vi "__move_motor2.vi"(3 "Moving distance":dbl=-50.0, 5 "motor setup":T1={"Axis"=0, "ID"=0, "HIspeed"=100.0, "LOspeed"=100.0, "ACCEL(ms)"=100.0, "Sratio"=50.0, "free ride"=TRUE, "string"="DSB HOT/COLD"}) -> (0 "error out":errorcluster, 2 "counter":dbl)   [LabVIEW 2017]
panel:
  in  "Ball":bool
  in  "Mcsd":refnum<k7>(container)
  # "<= HOT = reset to 0 and reset"
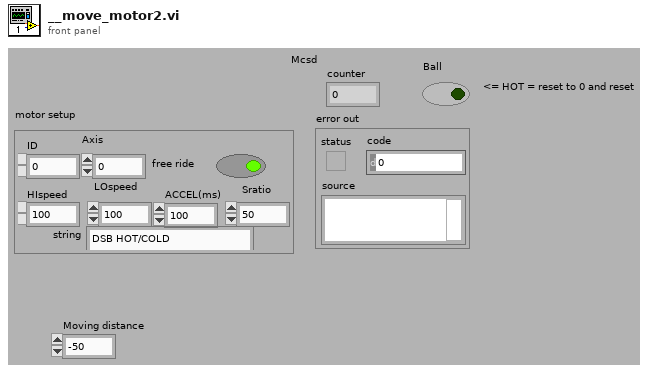
[diagram p1: front panel]
types:
  T1 = cluster{"Axis":i16, "ID":i16, "HIspeed":dbl, "LOspeed":dbl, "ACCEL(ms)":dbl, "Sratio":dbl, "free ride":bool, "string":string}
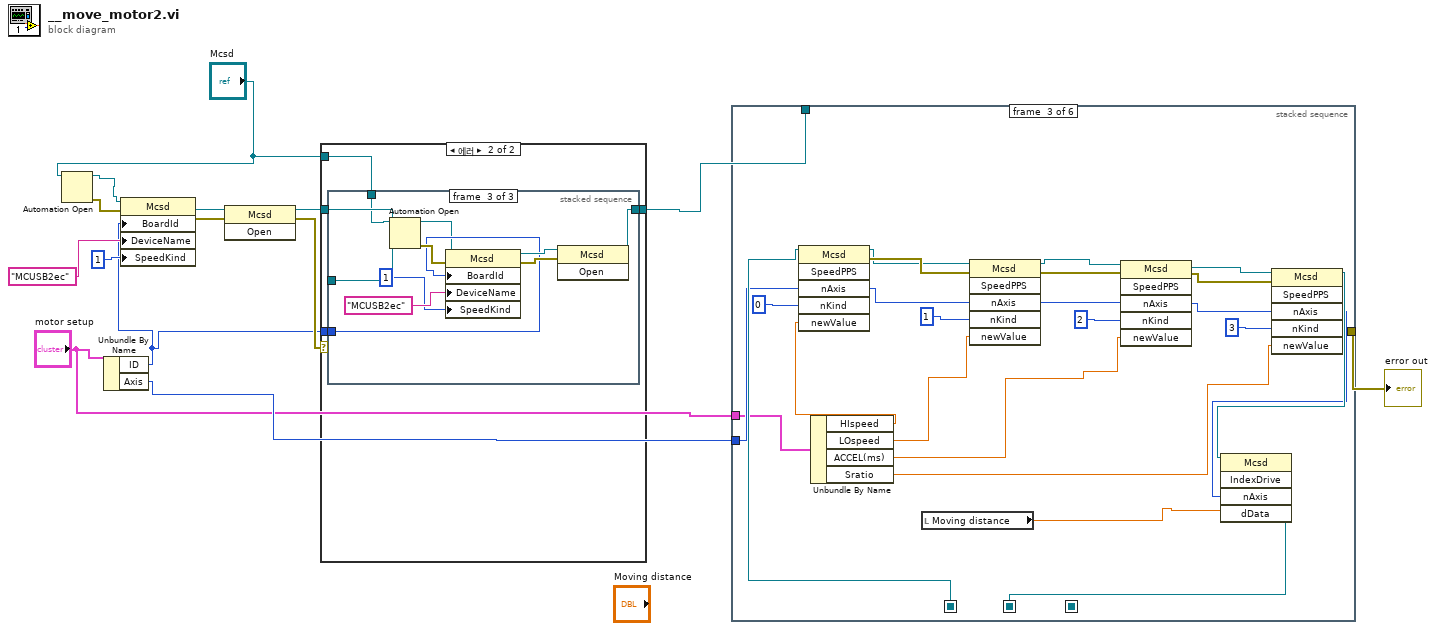
[diagram p0: block diagram]
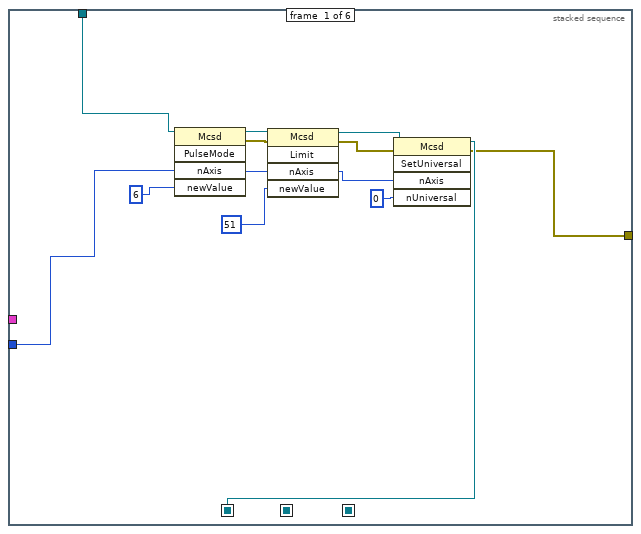
[diagram p2: hidden frame]
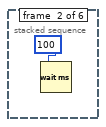
[diagram p3: hidden frame]
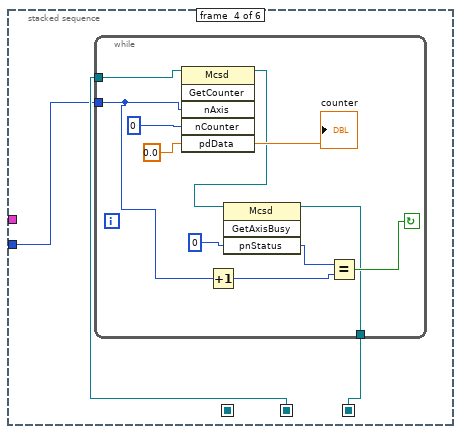
[diagram p4: hidden frame]
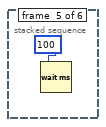
[diagram p5: hidden frame]
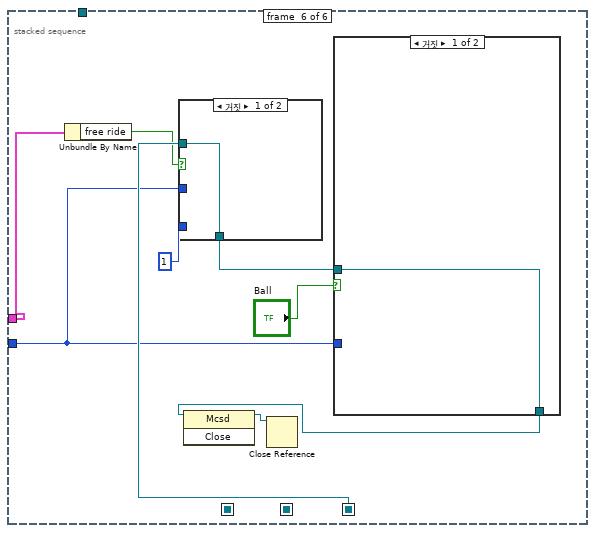
[diagram p6: hidden frame]
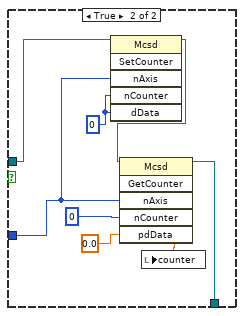
[diagram p7: hidden frame]
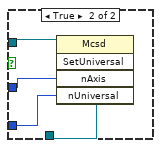
[diagram p8: hidden frame]
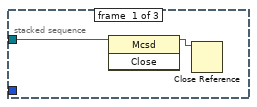
[diagram p10: hidden frame]
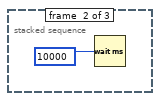
[diagram p11: hidden frame]
diagram:
  n1 = Automation Open(Automation Refnum="Mcsd") -> (Automation Refnum=w12:refnum<k7>, error out=w14:errorcluster)  [unwired: 3 in]
  n2 = Unbundle By Name("motor setup") -> ("ID"=w2:i16, "Axis"=w11:i16)
  n3 = property class="Mcsd"(reference=w12, error in=w14, "BoardId"=w2, "DeviceName"="MCUSB2ec", "SpeedKind"=1) -> (reference out=w9:refnum<k7>, error out=w13:errorcluster)
  n4 = invoke class="Mcsd" method="Open"(reference=w9, error in=w13) -> (reference out=w4:refnum<k7>, error out=w6:errorcluster)  [unwired: 1 in, 1 out]
  n5 = case shown="에러" w6 {
    tunnel: [w15 w16] -> w5
    tunnel: w4 -> [w15 w19]
    tunnel: w2 -> [_ w18]
    tunnel: "Mcsd" -> [_ w17]
    frame No Error {
    }
    frame Error {
      n6 = stacked-sequence {
        tunnel: w19 -> [w20 _ _]
        tunnel: w18 -> [_ _ w26]
        tunnel: w17 -> [_ _ w25]
        tunnel: [_ _ w24] -> w16
        frame #0 {
          n7 = invoke class="Mcsd" method="Close"(reference=w20) -> (reference out=w21:refnum<k7>)  [unwired: 2 in, 2 out]
          n8 = Close Reference(reference=w21) -> ()  [unwired: 1 in, 1 out]
        }
        frame #1 {
          n9 = Wait (ms)(milliseconds to wait=10000) -> ()  [unwired: 1 out]
        }
        frame #2 {
          n10 = Automation Open(Automation Refnum=w25) -> (Automation Refnum=w23:refnum<k7>, error out=w31:errorcluster)  [unwired: 3 in]
          n11 = property class="Mcsd"(reference=w23, error in=w31, "BoardId"=w26, "DeviceName"="MCUSB2ec", "SpeedKind"=1) -> (reference out=w29:refnum<k7>, error out=w30:errorcluster)
          n12 = invoke class="Mcsd" method="Open"(reference=w29, error in=w30) -> (reference out=w24:refnum<k7>)  [unwired: 1 in, 2 out]
        }
      }
    }
  }
  n13 = stacked-sequence {
    seq-local: [w43 _ _ _ _ _] -> [_ _ w54 _ _ _]
    seq-local: [_ _ w69 _ _ _] -> [_ _ _ w72 _ _]
    seq-local: [_ _ _ w70 _ _] -> [_ _ _ _ _ w91]
    tunnel: w5 -> [w41 _ _ _ _ _]
    tunnel: w11 -> [w39 _ w53 w71 _ w86]
    tunnel: [w42 _ _ _ _ _] -> w3
    tunnel: "motor setup" -> [_ _ w51 _ _ w90]
    frame #0 {
      n14 = invoke class="Mcsd" method="PulseMode"(reference=w41, "nAxis"=w39, "newValue"=6) -> (reference out=w38:refnum<k7>, error out=w37:errorcluster, "nAxis"=w33:i16)  [unwired: 2 in, 2 out]
      n15 = invoke class="Mcsd" method="Limit"(reference=w38, error in=w37, "nAxis"=w33, "newValue"=51) -> (reference out=w35:refnum<k7>, error out=w36:errorcluster, "nAxis"=w34:i16)  [unwired: 1 in, 2 out]
      n16 = invoke class="Mcsd" method="SetUniversal"(reference=w35, error in=w36, "nAxis"=w34, "nUniversal"=0) -> (reference out=w43:refnum<k7>, error out=w42:errorcluster)  [unwired: 1 in, 3 out]
    }
    frame #1 {
      n17 = Wait (ms)(milliseconds to wait=100) -> ()  [unwired: 1 out]
    }
    frame #2 {
      n18 = Unbundle By Name(w51) -> ("HIspeed"=w50:dbl, "LOspeed"=w49:dbl, "ACCEL(ms)"=w48:dbl, "Sratio"=w47:dbl)
      n19 = invoke class="Mcsd" method="SpeedPPS"(reference=w54, "nAxis"=w53, "nKind"=0, "newValue"=w50) -> (reference out=w58:refnum<k7>, error out=w66:errorcluster, "nAxis"=w63:i16)  [unwired: 2 in, 3 out]
      n20 = local read "Moving distance"() -> (w46:dbl)
      n21 = invoke class="Mcsd" method="SpeedPPS"(reference=w58, error in=w66, "nAxis"=w63, "nKind"=1, "newValue"=w49) -> (reference out=w60:refnum<k7>, error out=w67:errorcluster, "nAxis"=w64:i16)  [unwired: 1 in, 3 out]
      n22 = invoke class="Mcsd" method="SpeedPPS"(reference=w60, error in=w67, "nAxis"=w64, "nKind"=2, "newValue"=w48) -> (reference out=w62:refnum<k7>, error out=w68:errorcluster, "nAxis"=w65:i16)  [unwired: 1 in, 3 out]
      n23 = invoke class="Mcsd" method="SpeedPPS"(reference=w62, error in=w68, "nAxis"=w65, "nKind"=3, "newValue"=w47) -> (reference out=w55:refnum<k7>, "nAxis"=w52:i16)  [unwired: 1 in, 4 out]
      n24 = invoke class="Mcsd" method="IndexDrive"(reference=w55, "nAxis"=w52, "dData"=w46) -> (reference out=w69:refnum<k7>)  [unwired: 2 in, 4 out]
    }
    frame #3 {
      n25 = while {
        tunnel: w72 -> [w80]
        tunnel: w71 -> [w74]
        tunnel: [w73] -> w70
        stop <- w75 continue-if-true
        n26 = invoke class="Mcsd" method="GetCounter"(reference=w80, "nAxis"=w74, "nCounter"=0, "pdData"=0.0) -> (reference out=w78:refnum<k7>, "pdData"=→"counter":dbl)  [unwired: 2 in, 4 out]
        n27 = Increment(x=w74) -> (x+1=w76:i16)
        n28 = invoke class="Mcsd" method="GetAxisBusy"(reference=w78, "pnStatus"=0) -> (reference out=w73:refnum<k7>, "pnStatus"=w77:i16)  [unwired: 2 in, 2 out]
        n29 = Equal?(x=w77, y=w76) -> (x = y?=w75:bool)
      }
    }
    frame #4 {
      n30 = Wait (ms)(milliseconds to wait=100) -> ()  [unwired: 1 out]
    }
    frame #5 {
      n31 = Unbundle By Name(w90) -> ("free ride"=w89:bool)
      n32 = case shown="거짓" w89 {
        tunnel: 1 -> [_ w107]
        tunnel: [w103 w106] -> w87
        tunnel: w91 -> [w103 w104]
        tunnel: w86 -> [_ w105]
        frame False {
        }
        frame True {
          n33 = invoke class="Mcsd" method="SetUniversal"(reference=w104, "nAxis"=w105, "nUniversal"=w107) -> (reference out=w106:refnum<k7>)  [unwired: 2 in, 4 out]
        }
      }
      n34 = case shown="거짓" "Ball" {
        tunnel: w87 -> [w94 w98]
        tunnel: w86 -> [_ w97]
        tunnel: [w94 w95] -> w85
        frame False {
        }
        frame True {
          w99 = 0
          n35 = invoke class="Mcsd" method="SetCounter"(reference=w98, "nAxis"=w97, "nCounter"=w99, "dData"=w99) -> (reference out=w96:refnum<k7>)  [unwired: 2 in, 5 out]
          n36 = invoke class="Mcsd" method="GetCounter"(reference=w96, "nAxis"=w97, "nCounter"=0, "pdData"=0.0) -> (reference out=w95:refnum<k7>, "pdData"=w100:dbl)  [unwired: 2 in, 4 out]
          n37 = local write "counter"(w100) -> ()
        }
      }
      n38 = invoke class="Mcsd" method="Close"(reference=w85) -> (reference out=w92:refnum<k7>)  [unwired: 2 in, 2 out]
      n39 = Close Reference(reference=w92) -> ()  [unwired: 1 in, 1 out]
    }
  }
  "error out" <- w3
